vi "SPIRxRead.vi"(8 "error in (no error)":errorcluster caption="错误输入（无错误）", 10 "length":i32=256, 11 "handle":u64) -> (0 "error out":errorcluster caption="错误输出", 1 "rgRX":u8[](array[numeric]), 2 "function return":i32, 3 "handle out":u64, 4 "rxcount out":i32)   [LabVIEW 2018]
doc: "Read SPI datas"
uses:
  InstrumentsPlayground.lvlib
panel:
  out "fParity out":i32
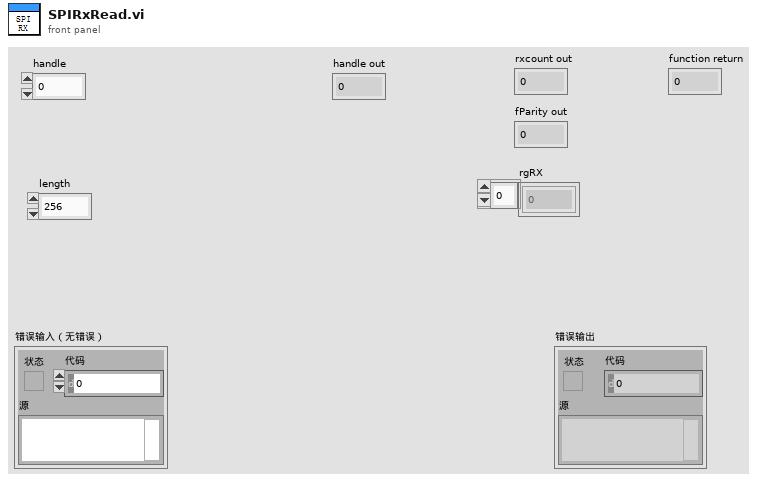
[diagram p1: front panel]
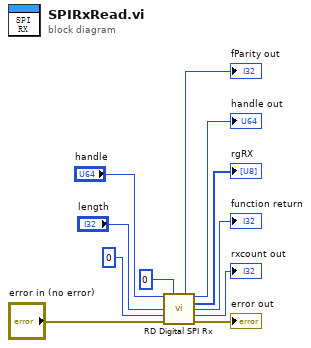
[diagram p0: block diagram]
diagram:
  n1 = call "RD Digital SPI Rx.vi"("handle"="handle", "fParity"=0, "length"="length", "rxcount"=0, "error in (no error)"="error in (no error)") -> ("fParity out"=→"fParity out":i32, "handle out"=→"handle out":u64, "rgRX out"=→"rgRX":u8[], "function return"=→"function return":i32, "rxcount out"=→"rxcount out":i32, "error out"=→"error out":errorcluster)  [unwired: 5 in]
